vi "FdxCmdTxUDPGetStatusCvi.vi"(8 "error in":errorcluster, 10 "UdpHandle":u32, 11 "InstrumentHandle":u32) -> (0 "error out":errorcluster, 1 "CurrentIndex":u32, 2 "UdpHandleOut":u32, 3 "InstrumentHandle":u32, 4 "IndexCycleCount":u32, 5 "MsgCount":u32)   [LabVIEW 2020, in "AIM664LV.lvlib"]
doc: "This function is used to retrieve the status of the specified UDP transmit port."
uses:
  AIM664LV.lvlib
  AFDX_LibraryAdmin/FdxGlobalDllPath.vi
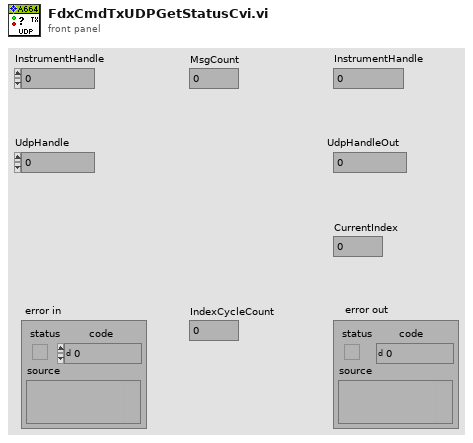
[diagram p1: front panel]
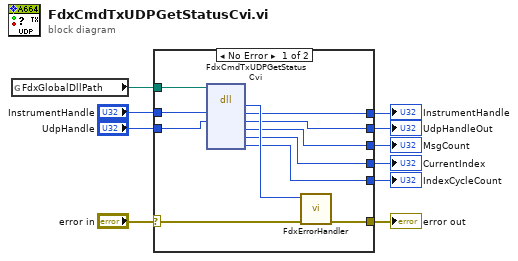
[diagram p0: block diagram]
diagram:
  n1 = global read "FdxGlobalDllPath.vi" "FdxGlobalDllPath"() -> (w8:path)
  n2 = case shown="No Error" "error in" {
    selector: "error in" -> [w20 w24]
    tunnel: [w21 w24] -> w10
    tunnel: w8 -> [w18 _]
    tunnel: "InstrumentHandle" -> [w17 w23]
    tunnel: [w16 w23] -> w6
    tunnel: "UdpHandle" -> [w15 w22]
    tunnel: [w14 _] -> w4
    tunnel: [w13 _] -> w3
    tunnel: [w12 _] -> w2
    tunnel: [w11 w22] -> w1
    frame No Error {
      n3 = dll-call lib="aim_fdx.19.dll" fn="FdxCmdTxUDPGetStatusCvi"(path in=w18, "InstrumentHandle"=w17, "UdpHandle"=w15) -> ("status"=w19:i32, "InstrumentHandle"=w16:u32, "UdpHandle"=w11:u32, "MsgCount"=w12:u32, "CurrentIndex"=w13:u32, "IndexCycleCount"=w14:u32)  [unwired: 2 in, 5 out]
      n4 = call "FdxErrorHandler.vi"("error in"=w20, "AIM Error"=w19) -> ("error out"=w21:errorcluster)  [unwired: 9 in]
    }
    frame Error {
    }
  }
  "error out" <- w10
  "InstrumentHandle" <- w6
  "MsgCount" <- w2
  "CurrentIndex" <- w3
  "IndexCycleCount" <- w4
  "UdpHandleOut" <- w1
